vi "Voice Level Controls.vi"(8 "error in":errorcluster, 11 "MIDI Controls in":variant) -> (0 "error out":errorcluster, 2 "Voice Level Controls out":variant)   [LabVIEW 2014, in "mySynthesizer.lvlib" / "Voice Level Controls.lvlib"]
uses:
  Voice Level Controls.lvlib
panel:
  in  "error in (no error)":errorcluster
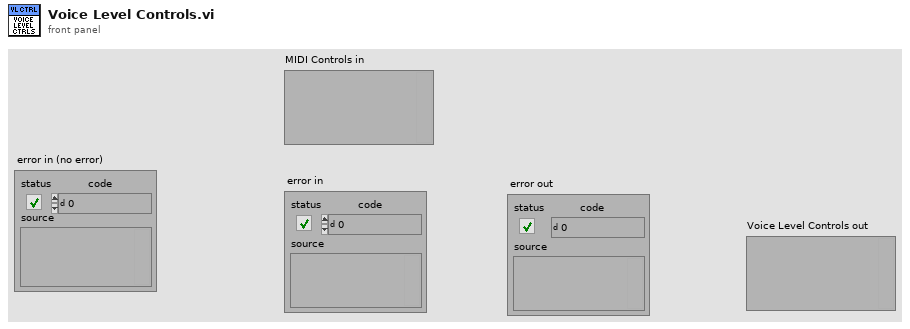
[diagram p1: front panel]
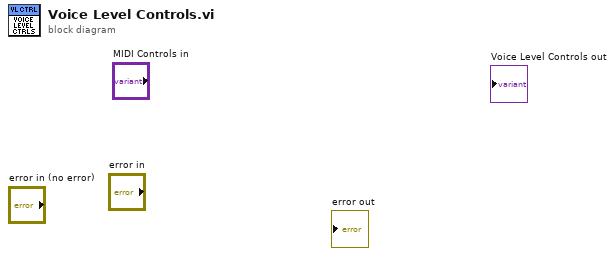
[diagram p0: block diagram]
diagram:
